vi "GUI-Get all FP Ctrl & Indi Label and Ref.vi"(11 "Respected VI Ref":refnum<vi>) -> (2 "All Object Label":string[](array[string]), 3 "All Object Ref":refnum<vi>[](array[refnum]))   [LabVIEW 2024]
panel:
  out "error out":errorcluster
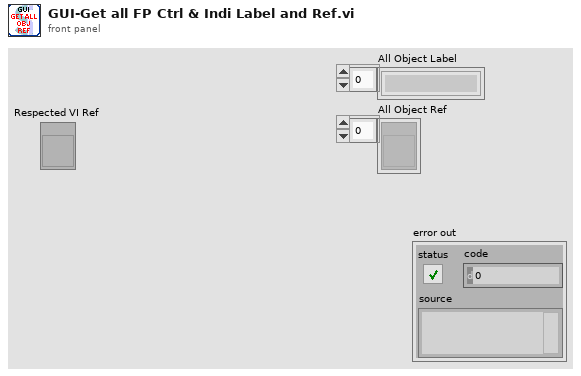
[diagram p1: front panel]
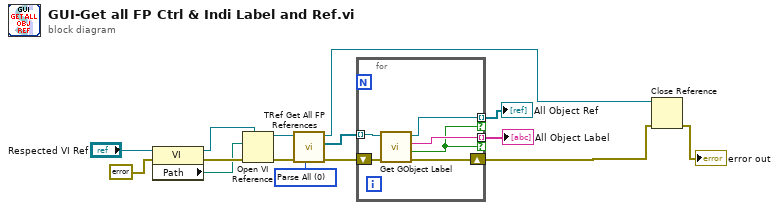
[diagram p0: block diagram]
diagram:
  w15 = u16 0 items=["Parse All", "Parse Tabs Only"] ("Parsing Rule")
  n1 = property class="VI"(reference="Respected VI Ref", error in=errorcluster {"status"=FALSE, "code"=0, "source"=""} ("error in (no error)")) -> (reference out=w14:refnum<vi>, error out=w13:errorcluster, "Path"=w12:path)
  n2 = Open VI Reference(type specifier VI Refnum (for type only)=w14, vi path=w12, error in (no error)=w13) -> (vi reference=w11:refnum<vi>, error out=w10:errorcluster)  [unwired: 3 in]
  n3 = call <vilib>:"TRef Get All FP References.vi"("Parsing Rule"=w15, "error in (no error)"=w10, "VI Refnum"=w11) -> ("error out"=w8:errorcluster, "All FP Objects"=w7:refnum<vi>[], "dup VI Refnum"=w3:refnum<vi>)  [unwired: 4 in, 2 out]
  n4 = for {
    tunnel: w7 -> [w20] mode=indexing
    shift-right: [w18] -> w2
    shift-left: w8 -> [w21]
    tunnel: [w19] -> w4 mode=indexing if=w16
    tunnel: [w17] -> w5 mode=indexing if=w16
    n5 = call <vilib>:"Get GObject Label.vi"("error in (no error)"=w21, "GObject"=w20) -> ("error out"=w18:errorcluster, "Object Has Label?"=w16:bool, "Object Label"=w17:string, "dup GObject"=w19:refnum<vi>)  [unwired: 5 in, 1 out]
  }
  "All Object Label" <- w5
  "All Object Ref" <- w4
  n6 = Close Reference(reference=w3, error in (no error)=w2) -> (error out=→"error out":errorcluster)
